vi "Finish.vi"   [LabVIEW 2018]
doc: "This VI is called just before exiting. It is expected to close I/O refnum, save collected data, etc."
uses:
  Typedefs/typedef_enum_refnums.ctl
  <vilib>/Rock Robotics/WPI/Utilities/WPI_GetSetVariantRefNum.vi
types:
  T1 = typedef "typedef_enum_refnums.ctl" = enum16{"Joy_L", "Joy_R", "Drive_Motors", "Intake_Motor", "Wrist_Solenoid", "Hatch_Solenoid", "Compressor", "Lift_Motor", "Lift_Motor_2", "Gyro", "Drive_Enc_L", "Drive_Enc_R", "Lift_Lower_Limit", "Lift_Upper_Limit", "Ball_Switch", "Jump_Solenoid"}
  T2 = typedef "WPI_JoystickDevRef.ctl" = cluster{"Device":T3}
  T3 = typedef "WPI_JoystickDeviceEnum.ctl" = enum16{"USB 0", "USB 1", "USB 2", "USB 3", "USB 4", "USB 5"}
  T4 = typedef "WPI_RobotDriveDevRef.ctl" = cluster{"DevStatus":errorcluster, "Motors[]":T5[], "Square Inputs":bool, "Max Output":dbl}
  T5 = typedef "WPI_MotorControlDeviceRef.ctl" = cluster{"DeviceStatus":errorcluster, "Type":T6, "PWM":cluster{"PWM Channel":T7, "DeadBand":T8}, "CAN":cluster{"Device Number":u8, "SetOutput VI Ref":variant, "GetOutput VI Ref":variant, "Enable VI Ref":variant, "Disable VI Ref":variant, "Data":variant}, "Invert":bool, "DIO PWM":cluster{"PWM \"Enable\" Channel":T7, "DIOChannel":T9, "PWM Rate":dbl}}
  T6 = typedef "WPI_MotorControlType.ctl" = enum16{"PWM", "CAN", "DIO PWM"}
  T7 = typedef "FPGA_DIOPWMChannel.ctl" = enum8{"PWM 0", "PWM 1", "PWM 2", "PWM 3", "PWM 4", "PWM 5", "PWM 6", "PWM 7", "PWM 8", "PWM 9", "PWM MXP 0", "PWM MXP 1", "PWM MXP 2", "PWM MXP 3", "PWM MXP 4", "PWM MXP 5", "PWM MXP 6", "PWM MXP 7", "PWM MXP 8", "PWM MXP 9", "Invalid"}
  T8 = typedef "WPI_PWMDeadband.ctl" = cluster{"Name":string, "maxPositivePwm":i32, "minPositivePwm":i32, "centerPwm":i32, "maxNegativePwm":i32, "minNegativePwm":i32, "angularRange":u16}
  T9 = typedef "FPGA_DIOChannel.ctl" = enum8{"DIO 0", "DIO 1", "DIO 2", "DIO 3", "DIO 4", "DIO 5", "DIO 6", "DIO 7", "DIO 8", "DIO 9", "DIO MXP 0", "DIO MXP 1", "DIO MXP 2", "DIO MXP 3", "DIO MXP 4", "DIO MXP 5", "DIO MXP 6", "DIO MXP 7", "DIO MXP 8", "DIO MXP 9", "DIO MXP 10", "DIO MXP 11", "DIO MXP 12", "DIO MXP 13", "DIO MXP 14", "DIO MXP 15", "SPI Port CS1", "SPI Port CS2", "SPI Port CS3", "SPI Port MISO", "SPI Port MOSI", "Invalid"}
  T10 = typedef "WPI_SolenoidDevRef.ctl" = cluster{"DevStatus":errorcluster, "Pneumatics Control Module":u8, "Forward Solenoid Channel":T11, "Reverse Solenoid Channel":T11}
  T11 = typedef "WPI_SolenoidChannel.ctl" = enum8{"Solenoid 0", "Solenoid 1", "Solenoid 2", "Solenoid 3", "Solenoid 4", "Solenoid 5", "Solenoid 6", "Solenoid 7", "Invalid"}
  T12 = typedef "WPI_CompressorDevRef.ctl" = cluster{"DevStatus":errorcluster, "Pneumatics Control Module":u8}
  T13 = typedef "WPI_SwitchDevRef.ctl" = cluster{"DevStatus":errorcluster, "DIO Channel":T9, "CntIndex":T14, "Normally Closed":bool}
  T14 = typedef "FPGA_CounterCtrSystemIndex.ctl" = enum8{"Ctr 0", "Ctr 1", "Ctr 2", "Ctr 3", "Ctr 4", "Ctr 5", "Ctr 6", "Ctr 7", "Invalid"}
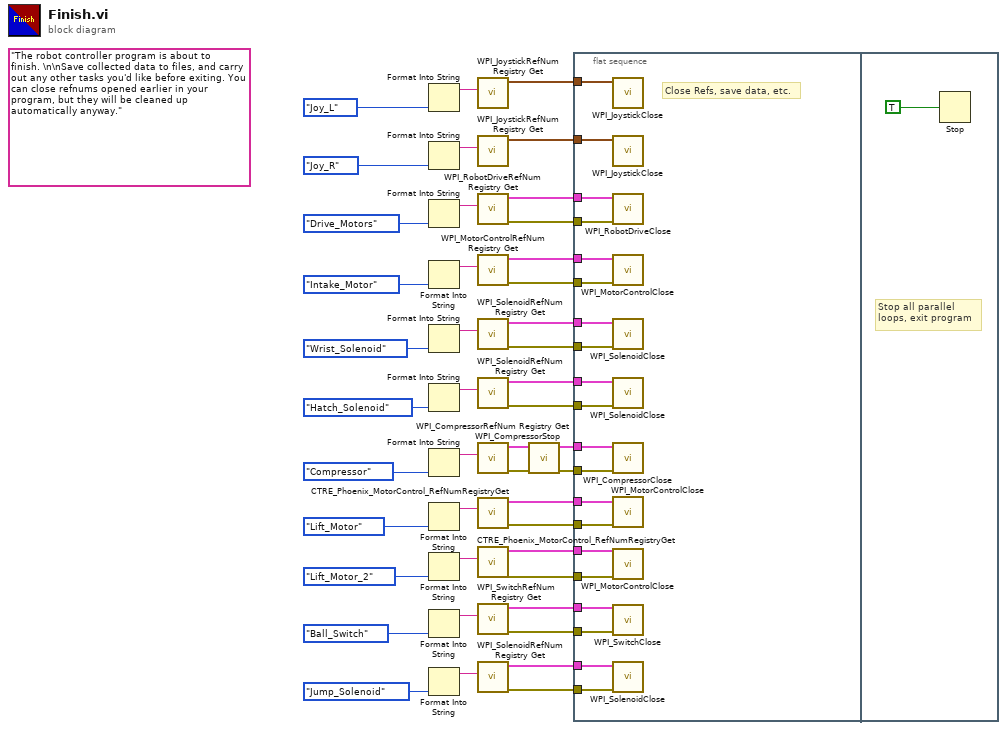
[diagram p0: block diagram]
diagram:
  (unwired) "The robot controller program is about to finish. \n\nSave collected data to files, and carry out any other tasks you'd like before exiting. You can close refnums opened earlier in your program, but they will be cleaned up automatically anyway."
  n1 = Format Into String(typedef_enum_refnums."Joy_L" ("Enum")) -> (resulting string=w33:string)  [unwired: 3 in, 1 out]
  n2 = Format Into String(typedef_enum_refnums."Joy_R" ("Enum")) -> (resulting string=w31:string)  [unwired: 3 in, 1 out]
  n3 = Format Into String(typedef_enum_refnums."Drive_Motors" ("Enum")) -> (resulting string=w35:string)  [unwired: 3 in, 1 out]
  n4 = Format Into String(typedef_enum_refnums."Intake_Motor" ("Enum")) -> (resulting string=w37:string)  [unwired: 3 in, 1 out]
  n5 = Format Into String(typedef_enum_refnums."Wrist_Solenoid" ("Enum")) -> (resulting string=w20:string)  [unwired: 3 in, 1 out]
  n6 = Format Into String(typedef_enum_refnums."Hatch_Solenoid" ("Enum")) -> (resulting string=w18:string)  [unwired: 3 in, 1 out]
  n7 = Format Into String(typedef_enum_refnums."Compressor" ("Enum")) -> (resulting string=w24:string)  [unwired: 3 in, 1 out]
  n8 = Format Into String(typedef_enum_refnums."Lift_Motor" ("Enum")) -> (resulting string=w6:string)  [unwired: 3 in, 1 out]
  n9 = Format Into String(typedef_enum_refnums."Lift_Motor_2" ("Enum")) -> (resulting string=w3:string)  [unwired: 3 in, 1 out]
  n10 = Format Into String(typedef_enum_refnums."Ball_Switch" ("Enum")) -> (resulting string=w9:string)  [unwired: 3 in, 1 out]
  n11 = Format Into String(typedef_enum_refnums."Jump_Solenoid" ("Enum")) -> (resulting string=w12:string)  [unwired: 3 in, 1 out]
  n12 = call <vilib>:"WPI_JoystickRefNum Registry Get.vi"("refnum name"=w33) -> ("JoystickDevRef"=w43:T2)  [unwired: 1 in, 9 out]
  n13 = call <vilib>:"WPI_JoystickRefNum Registry Get.vi"("refnum name"=w31) -> ("JoystickDevRef"=w30:T2)  [unwired: 1 in, 9 out]
  n14 = call <vilib>:"WPI_RobotDriveRefNum Registry Get.vi"("refnum name"=w35) -> ("error out"=w40:errorcluster, "RobotDriveDevRef"=w44:T4)  [unwired: 1 in, 8 out]
  n15 = call <vilib>:"WPI_MotorControlRefNum Registry Get.vi"("refnum name"=w37) -> ("error out"=w41:errorcluster, "MotorControlDevRef"=w42:T5)  [unwired: 9 in]
  n16 = call <vilib>:"WPI_SolenoidRefNum Registry Get.vi"("refnum name"=w20) -> ("error out"=w22:errorcluster, "SolenoidDevRef"=w23:T10)  [unwired: 9 in]
  n17 = call <vilib>:"WPI_SolenoidRefNum Registry Get.vi"("refnum name"=w18) -> ("error out"=w17:errorcluster, "SolenoidDevRef"=w16:T10)  [unwired: 9 in]
  n18 = call <vilib>:"WPI_CompressorRefNum Registry Get.vi"("refnum name"=w24) -> ("error out"=w27:errorcluster, "CompressorDevRef"=w26:T12)  [unwired: 9 in]
  n19 = call <vilib>:"CTRE_Phoenix_MotorControl_RefNumRegistryGet.vi"("refnum name"=w6) -> ("error out"=w4:errorcluster, "PhoenixMotorControlDevRef"=w5:T5)  [unwired: 9 in]
  n20 = call <vilib>:"CTRE_Phoenix_MotorControl_RefNumRegistryGet.vi"("refnum name"=w3) -> ("error out"=w1:errorcluster, "PhoenixMotorControlDevRef"=w2:T5)  [unwired: 9 in]
  n21 = call <vilib>:"WPI_SwitchRefNum Registry Get.vi"("refnum name"=w9) -> ("error out"=w7:errorcluster, "SwitchDevRef"=w8:T13)  [unwired: 9 in]
  n22 = call <vilib>:"WPI_SolenoidRefNum Registry Get.vi"("refnum name"=w12) -> ("error out"=w10:errorcluster, "SolenoidDevRef"=w11:T10)  [unwired: 9 in]
  n23 = call <vilib>:"WPI_CompressorStop.vi"("error in (no error)"=w27, "CompressorDevRef"=w26) -> ("error out"=w28:errorcluster, "CompressorDevRef"=w29:T12)  [unwired: 8 in]
  n24 = flat-sequence {
    tunnel: w44 -> [w64]
    tunnel: w43 -> [w63]
    tunnel: w42 -> [w62]
    tunnel: w41 -> [w61]
    tunnel: w40 -> [w60]
    tunnel: w30 -> [w59]
    tunnel: w29 -> [w58]
    tunnel: w28 -> [w57]
    tunnel: w23 -> [w56]
    tunnel: w22 -> [w55]
    tunnel: w17 -> [w54]
    tunnel: w16 -> [w53]
    tunnel: w11 -> [w52]
    tunnel: w10 -> [w51]
    tunnel: w8 -> [w50]
    tunnel: w7 -> [w49]
    tunnel: w5 -> [w48]
    tunnel: w4 -> [w47]
    tunnel: w2 -> [w46]
    tunnel: w1 -> [w45]
    frame #0 {
      # "Close Refs, save data, etc."
      n25 = call <vilib>:"WPI_JoystickClose.vi"("JoystickDevRef"=w63) -> ()  [unwired: 11 out]
      n26 = call <vilib>:"WPI_JoystickClose.vi"("JoystickDevRef"=w59) -> ()  [unwired: 11 out]
      n27 = call <vilib>:"WPI_RobotDriveClose.vi"("error in (no error)"=w60, "RobotDriveDevRef"=w64) -> ()  [unwired: 10 out]
      n28 = call <vilib>:"WPI_MotorControlClose.vi"("error in"=w61, "MotorControlDevRef"=w62) -> ()  [unwired: 9 in, 1 out]
      n29 = call <vilib>:"WPI_SolenoidClose.vi"("error in (no error)"=w55, "SolenoidDevRef"=w56) -> ()  [unwired: 9 in, 1 out]
      n30 = call <vilib>:"WPI_SolenoidClose.vi"("error in (no error)"=w54, "SolenoidDevRef"=w53) -> ()  [unwired: 9 in, 1 out]
      n31 = call <vilib>:"WPI_CompressorClose.vi"("error in (no error)"=w57, "CompressorDevRef"=w58) -> ()  [unwired: 9 in, 1 out]
      n32 = call <vilib>:"WPI_MotorControlClose.vi"("error in"=w47, "MotorControlDevRef"=w48) -> ()  [unwired: 9 in, 1 out]
      n33 = call <vilib>:"WPI_MotorControlClose.vi"("error in"=w45, "MotorControlDevRef"=w46) -> ()  [unwired: 9 in, 1 out]
      n34 = call <vilib>:"WPI_SwitchClose.vi"("error in (no error)"=w49, "SwitchDevRef"=w50) -> ()  [unwired: 9 in, 1 out]
      n35 = call <vilib>:"WPI_SolenoidClose.vi"("error in (no error)"=w51, "SolenoidDevRef"=w52) -> ()  [unwired: 9 in, 1 out]
    }
    frame #1 {
      # "Stop all parallel\nloops, exit program"
      n36 = Stop(stop? (T)=TRUE ("Quit")) -> ()
    }
  }
